vi "_RUN_HVAC_PROJECT.vi"() -> ()   [LabVIEW 2011]
panel:
  in  "Tab Control":T1(tab)
  in  "Stop":bool
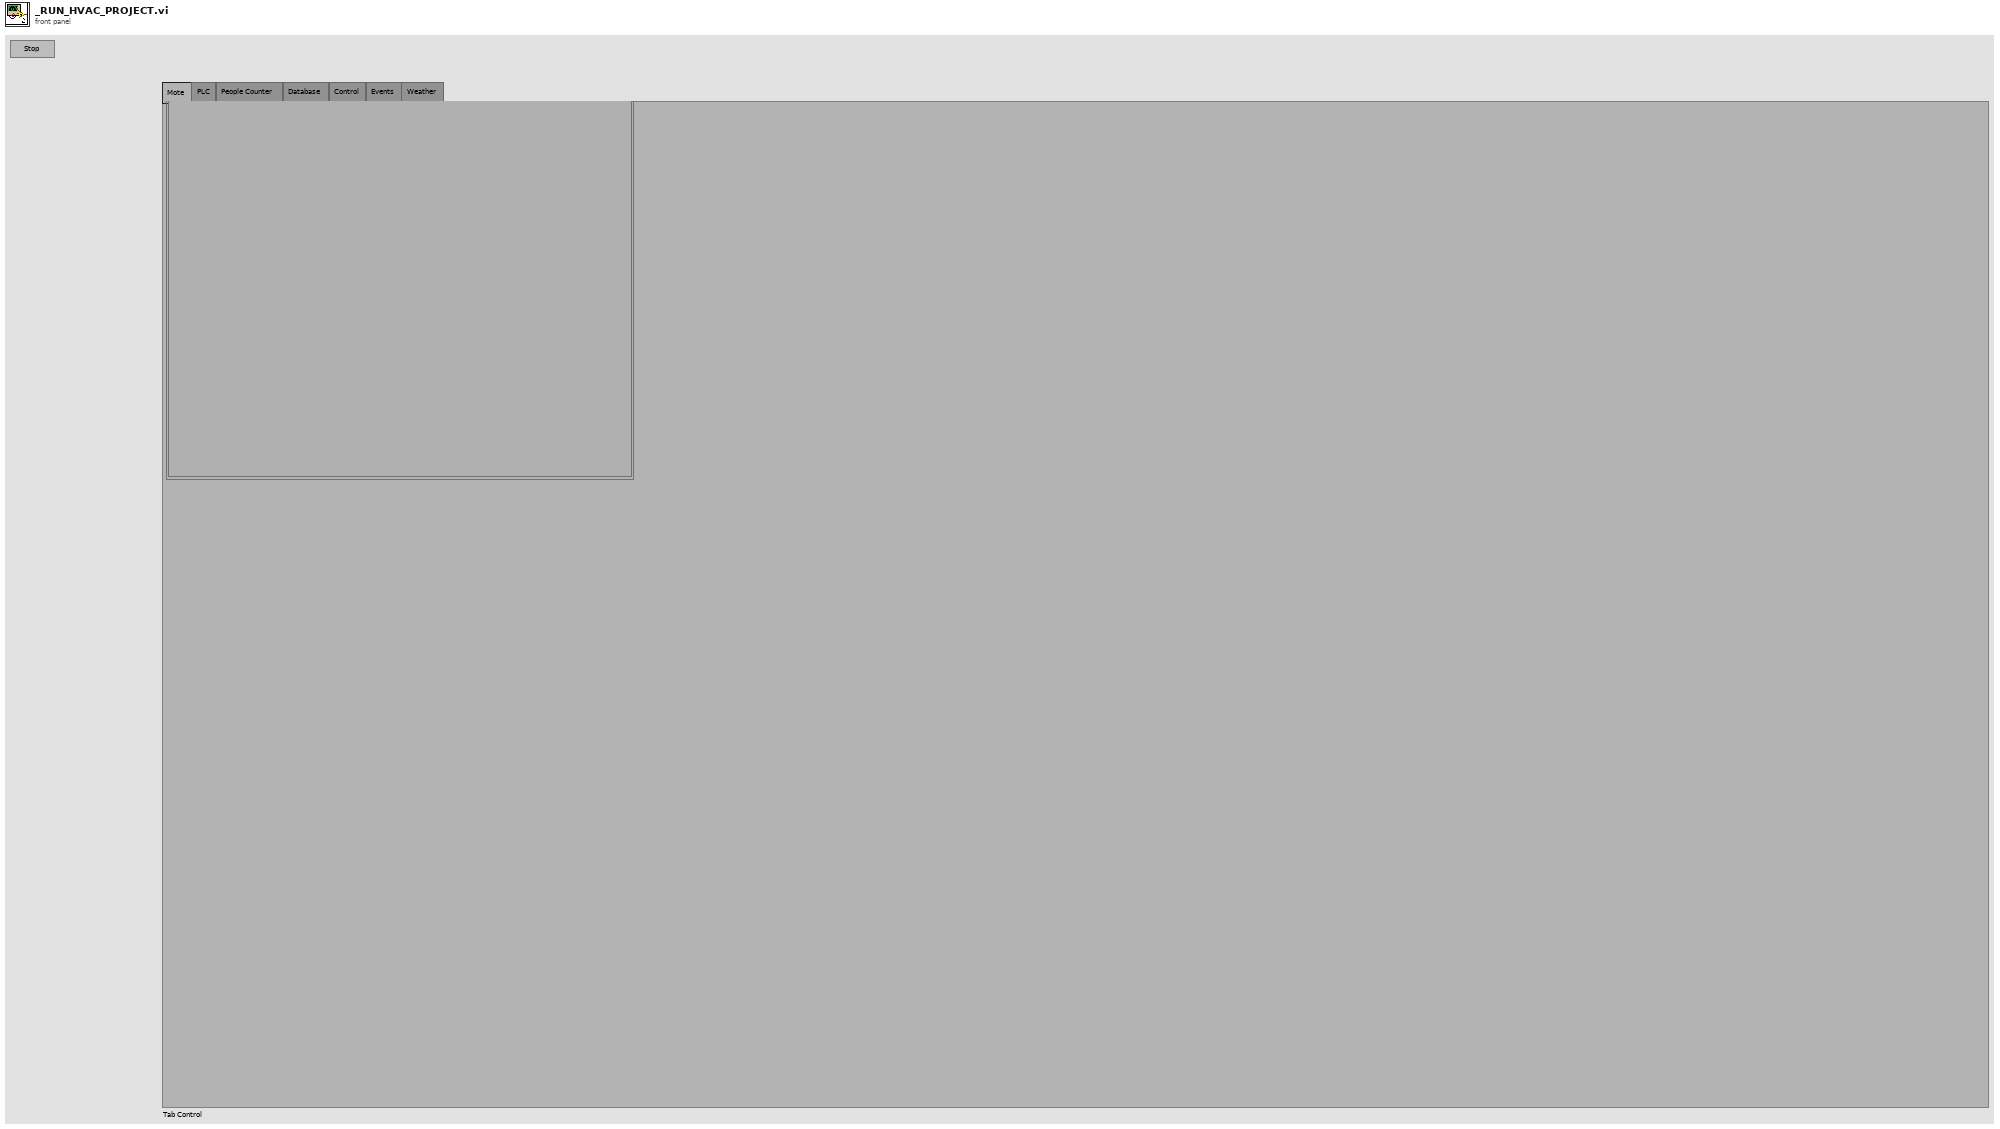
[diagram p1: front panel]
types:
  T1 = enum32{"Mote", "PLC", "People Counter", "Database", "Control", "Events", "Weather"}
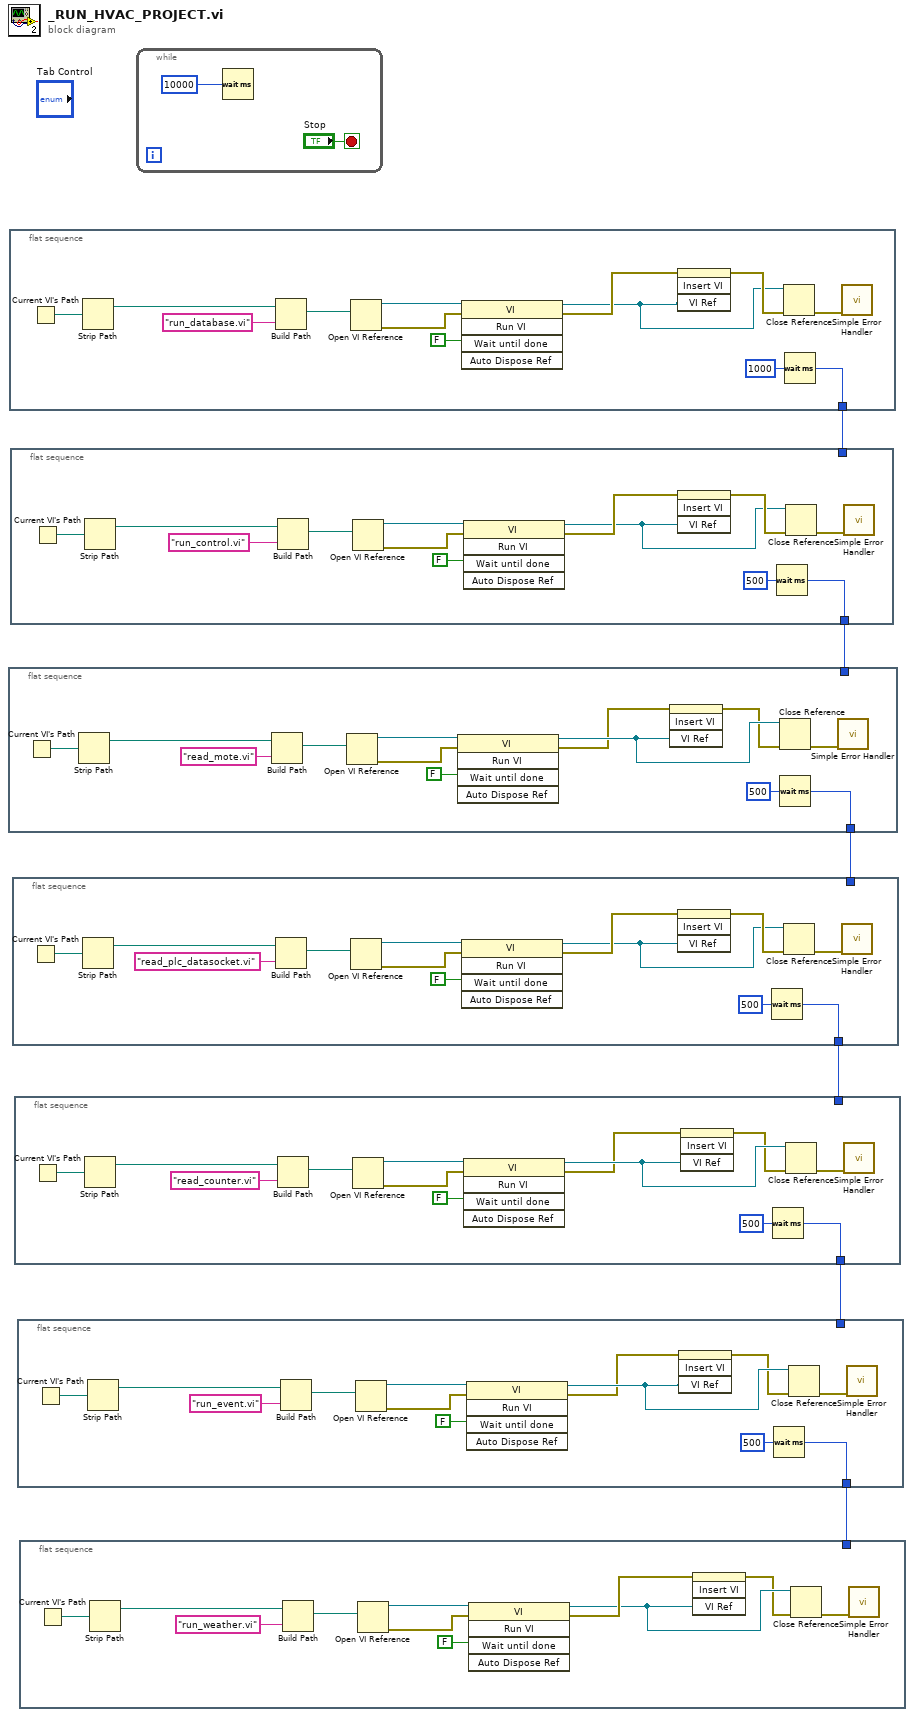
[diagram p0: block diagram]
diagram:
  n1 = flat-sequence {
    tunnel: [w7] -> w4
    tunnel: w5 -> [_]
    frame #0 {
      n2 = Current VI's Path() -> (path=w16:path)
      n3 = Strip Path(path=w16) -> (stripped path=w14:path)  [unwired: 1 out]
      n4 = Build Path(base path=w14, name or relative path="read_mote.vi") -> (appended path=w15:path)
      n5 = Open VI Reference(vi path=w15) -> (vi reference=w19:refnum<vi>, error out=w18:errorcluster)  [unwired: 5 in]
      n6 = invoke class="VI" method="Run VI"(reference=w19, error in=w18, "Wait until done"=FALSE) -> (reference out=w11:refnum<vi>, error out=w10:errorcluster)  [unwired: 2 in, 3 out]
      n7 = invoke class="SubPanel" method="Insert VI"(error in=w10, "VI Ref"=w11) -> (error out=w9:errorcluster)  [unwired: 2 in, 3 out]
      n8 = Close Reference(reference=w11, error in (no error)=w9) -> (error out=w13:errorcluster)
      n9 = Wait (ms)(milliseconds to wait=u32 500) -> (millisecond timer value=w7:u32)
      n10 = call <vilib>:"Simple Error Handler.vi"("error in (no error)"=w13) -> ()  [unwired: 4 in, 5 out]
    }
  }
  n11 = flat-sequence {
    tunnel: [w20] -> w6
    frame #0 {
      n12 = Current VI's Path() -> (path=w29:path)
      n13 = Strip Path(path=w29) -> (stripped path=w27:path)  [unwired: 1 out]
      n14 = Build Path(base path=w27, name or relative path="run_database.vi") -> (appended path=w28:path)
      n15 = Open VI Reference(vi path=w28) -> (vi reference=w32:refnum<vi>, error out=w31:errorcluster)  [unwired: 5 in]
      n16 = invoke class="VI" method="Run VI"(reference=w32, error in=w31, "Wait until done"=FALSE) -> (reference out=w22:refnum<vi>, error out=w23:errorcluster)  [unwired: 2 in, 3 out]
      n17 = invoke class="SubPanel" method="Insert VI"(error in=w23, "VI Ref"=w22) -> (error out=w24:errorcluster)  [unwired: 2 in, 3 out]
      n18 = Close Reference(reference=w22, error in (no error)=w24) -> (error out=w26:errorcluster)
      n19 = Wait (ms)(milliseconds to wait=u32 1000) -> (millisecond timer value=w20:u32)
      n20 = call <vilib>:"Simple Error Handler.vi"("error in (no error)"=w26) -> ()  [unwired: 4 in, 5 out]
    }
  }
  n21 = flat-sequence {
    tunnel: w6 -> [_]
    tunnel: [w33] -> w5
    frame #0 {
      n22 = Current VI's Path() -> (path=w41:path)
      n23 = Strip Path(path=w41) -> (stripped path=w43:path)  [unwired: 1 out]
      n24 = Build Path(base path=w43, name or relative path="run_control.vi") -> (appended path=w42:path)
      n25 = Open VI Reference(vi path=w42) -> (vi reference=w38:refnum<vi>, error out=w39:errorcluster)  [unwired: 5 in]
      n26 = invoke class="VI" method="Run VI"(reference=w38, error in=w39, "Wait until done"=FALSE) -> (reference out=w35:refnum<vi>, error out=w36:errorcluster)  [unwired: 2 in, 3 out]
      n27 = invoke class="SubPanel" method="Insert VI"(error in=w36, "VI Ref"=w35) -> (error out=w37:errorcluster)  [unwired: 2 in, 3 out]
      n28 = Wait (ms)(milliseconds to wait=u32 500) -> (millisecond timer value=w33:u32)
      n29 = Close Reference(reference=w35, error in (no error)=w37) -> (error out=w44:errorcluster)
      n30 = call <vilib>:"Simple Error Handler.vi"("error in (no error)"=w44) -> ()  [unwired: 4 in, 5 out]
    }
  }
  n31 = flat-sequence {
    tunnel: w4 -> [_]
    tunnel: [w46] -> w3
    frame #0 {
      n32 = Current VI's Path() -> (path=w54:path)
      n33 = Strip Path(path=w54) -> (stripped path=w56:path)  [unwired: 1 out]
      n34 = Build Path(base path=w56, name or relative path="read_plc_datasocket.vi") -> (appended path=w55:path)
      n35 = Open VI Reference(vi path=w55) -> (vi reference=w51:refnum<vi>, error out=w52:errorcluster)  [unwired: 5 in]
      n36 = invoke class="VI" method="Run VI"(reference=w51, error in=w52, "Wait until done"=FALSE) -> (reference out=w48:refnum<vi>, error out=w49:errorcluster)  [unwired: 2 in, 3 out]
      n37 = invoke class="SubPanel" method="Insert VI"(error in=w49, "VI Ref"=w48) -> (error out=w50:errorcluster)  [unwired: 2 in, 3 out]
      n38 = Wait (ms)(milliseconds to wait=u32 500) -> (millisecond timer value=w46:u32)
      n39 = Close Reference(reference=w48, error in (no error)=w50) -> (error out=w57:errorcluster)
      n40 = call <vilib>:"Simple Error Handler.vi"("error in (no error)"=w57) -> ()  [unwired: 4 in, 5 out]
    }
  }
  n41 = flat-sequence {
    tunnel: w3 -> [_]
    tunnel: [w59] -> w2
    frame #0 {
      n42 = Current VI's Path() -> (path=w67:path)
      n43 = Strip Path(path=w67) -> (stripped path=w69:path)  [unwired: 1 out]
      n44 = Build Path(base path=w69, name or relative path="read_counter.vi") -> (appended path=w68:path)
      n45 = Open VI Reference(vi path=w68) -> (vi reference=w64:refnum<vi>, error out=w65:errorcluster)  [unwired: 5 in]
      n46 = invoke class="VI" method="Run VI"(reference=w64, error in=w65, "Wait until done"=FALSE) -> (reference out=w63:refnum<vi>, error out=w62:errorcluster)  [unwired: 2 in, 3 out]
      n47 = invoke class="SubPanel" method="Insert VI"(error in=w62, "VI Ref"=w63) -> (error out=w61:errorcluster)  [unwired: 2 in, 3 out]
      n48 = Wait (ms)(milliseconds to wait=u32 500) -> (millisecond timer value=w59:u32)
      n49 = Close Reference(reference=w63, error in (no error)=w61) -> (error out=w70:errorcluster)
      n50 = call <vilib>:"Simple Error Handler.vi"("error in (no error)"=w70) -> ()  [unwired: 4 in, 5 out]
    }
  }
  n51 = flat-sequence {
    tunnel: w2 -> [_]
    tunnel: [w72] -> w1
    frame #0 {
      n52 = Current VI's Path() -> (path=w80:path)
      n53 = Strip Path(path=w80) -> (stripped path=w82:path)  [unwired: 1 out]
      n54 = Build Path(base path=w82, name or relative path="run_event.vi") -> (appended path=w81:path)
      n55 = Open VI Reference(vi path=w81) -> (vi reference=w77:refnum<vi>, error out=w78:errorcluster)  [unwired: 5 in]
      n56 = invoke class="VI" method="Run VI"(reference=w77, error in=w78, "Wait until done"=FALSE) -> (reference out=w76:refnum<vi>, error out=w75:errorcluster)  [unwired: 2 in, 3 out]
      n57 = invoke class="SubPanel" method="Insert VI"(error in=w75, "VI Ref"=w76) -> (error out=w74:errorcluster)  [unwired: 2 in, 3 out]
      n58 = Wait (ms)(milliseconds to wait=u32 500) -> (millisecond timer value=w72:u32)
      n59 = Close Reference(reference=w76, error in (no error)=w74) -> (error out=w83:errorcluster)
      n60 = call <vilib>:"Simple Error Handler.vi"("error in (no error)"=w83) -> ()  [unwired: 4 in, 5 out]
    }
  }
  n61 = flat-sequence {
    tunnel: w1 -> [_]
    frame #0 {
      n62 = Current VI's Path() -> (path=w91:path)
      n63 = Strip Path(path=w91) -> (stripped path=w93:path)  [unwired: 1 out]
      n64 = Build Path(base path=w93, name or relative path="run_weather.vi") -> (appended path=w92:path)
      n65 = Open VI Reference(vi path=w92) -> (vi reference=w88:refnum<vi>, error out=w89:errorcluster)  [unwired: 5 in]
      n66 = invoke class="VI" method="Run VI"(reference=w88, error in=w89, "Wait until done"=FALSE) -> (reference out=w86:refnum<vi>, error out=w87:errorcluster)  [unwired: 2 in, 3 out]
      n67 = invoke class="SubPanel" method="Insert VI"(error in=w87, "VI Ref"=w86) -> (error out=w85:errorcluster)  [unwired: 2 in, 3 out]
      n68 = Close Reference(reference=w86, error in (no error)=w85) -> (error out=w94:errorcluster)
      n69 = call <vilib>:"Simple Error Handler.vi"("error in (no error)"=w94) -> ()  [unwired: 4 in, 5 out]
    }
  }
  n70 = while {
    stop <- "Stop" stop-if-true
    n71 = Wait (ms)(milliseconds to wait=u32 10000) -> ()  [unwired: 1 out]
  }
